vi "Write Default Compression level.vi"(8 "error in (no error)":errorcluster, 10 "Default Compression level":i32=3, 11 "lvzstd in":refnum<class "lvzstd.lvclass">) -> (0 "error out":errorcluster, 3 "lvzstd out":refnum<class "lvzstd.lvclass">)   [LabVIEW 2020, in "lvzstd.lvlib" / "lvzstd.lvclass"]
uses:
  lvzstd.lvclass
  lvzstd.lvclass/lvzstd.ctl
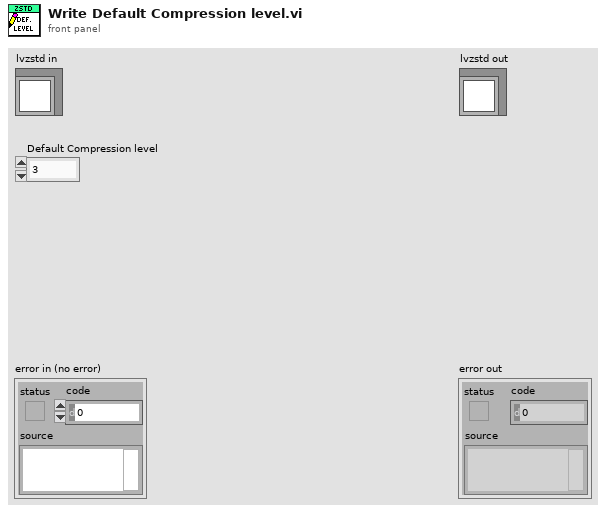
[diagram p1: front panel]
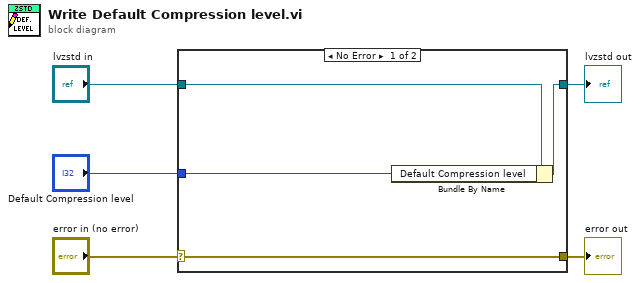
[diagram p0: block diagram]
diagram:
  n1 = case shown="No Error" "error in (no error)" {
    selector: "error in (no error)" -> [w9 w10]
    tunnel: [w9 w10] -> w4
    tunnel: [w7 w11] -> w2
    tunnel: "lvzstd in" -> [w8 w11]
    tunnel: "Default Compression level" -> [w6 _]
    frame No Error {
      n2 = Bundle By Name(cluster=w8, "Default Compression level"=w6) -> (w7:refnum<class "lvzstd.lvclass">)
    }
    frame Error {
    }
  }
  "error out" <- w4
  "lvzstd out" <- w2
